vi "Telescope Read Current Status.vi"(8 "error in (no error)":errorcluster, 11 "PRIME Telescope in":refnum<class "PRIME Telescope.lvclass">) -> (0 "error out":errorcluster, 1 "Raw Response":string, 2 "Telescope Status":T1, 3 "PRIME Telescope out":refnum<class "PRIME Telescope.lvclass">, 4 "Cmd Sent":string="A 001 004 009 018 020 017\r")   [LabVIEW 2024, in "PRIME Telescope.lvclass"]
uses:
  PRIME Telescope.lvclass
  Telescope cluster Status.ctl
  typedefs/CC cluster RA and DEC.ctl
  Telescope enum Status.ctl
  PRIME Telescope.lvclass/PRIME Telescope.ctl
  Telescope.lvclass
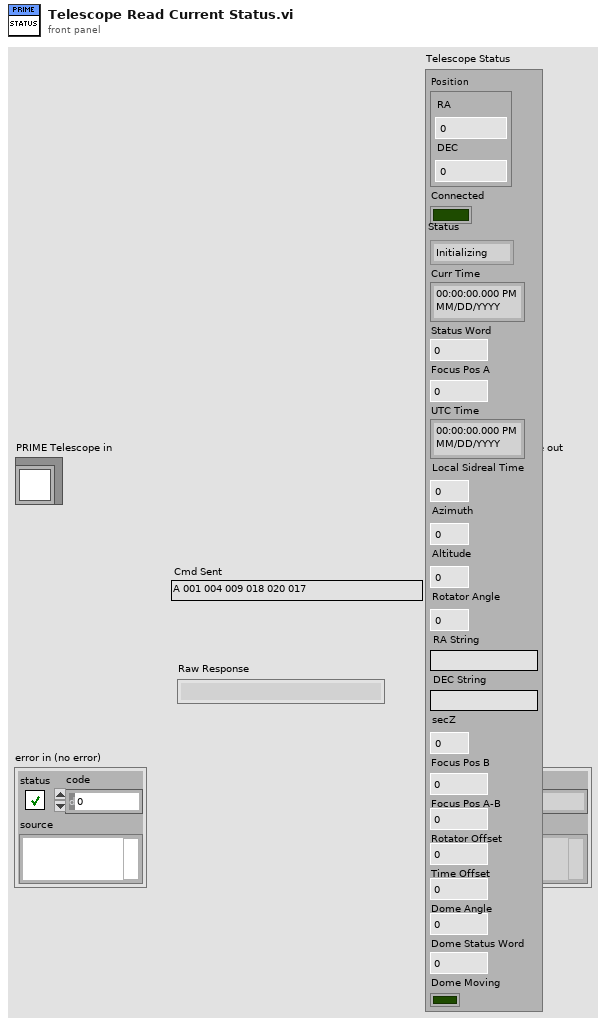
[diagram p1: front panel]
types:
  T1 = typedef "Telescope.lvclass/Telescope cluster Status.ctl" = cluster{"Position":T2, "Connected":bool, "Status":T3, "Curr Time":timestamp, "Status Word":u32, "Focus Pos A":dbl, "UTC Time":timestamp, "Local Sidreal Time":dbl, "Azimuth":dbl, "Altitude":dbl, "Rotator Angle":dbl, "RA String":string, "DEC String":string, "secZ":dbl, "Focus Pos B":dbl, "Focus Pos A-B":dbl, "Rotator Offset":dbl, "Time Offset":dbl, "Dome Angle":dbl, "Dome Status Word":u32, "Dome Moving":bool}
  T2 = typedef "CC cluster RA and DEC.ctl" = cluster{"RA":dbl, "DEC":dbl}
  T3 = typedef "Telescope.lvclass/Telescope enum Status.ctl" = enum16{"Initializing", "Ready", "Moving", "Focusing", "Error"}
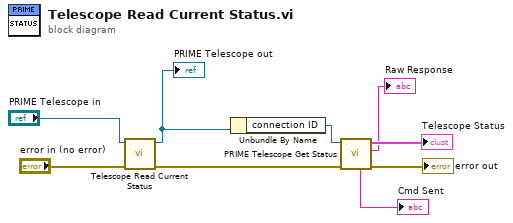
[diagram p0: block diagram]
diagram:
  n1 = call-parent "Telescope Read Current Status.vi"("error in (no error)"="error in (no error)", "Telescope in"="PRIME Telescope in") -> ("error out"=w5:errorcluster, "Telescope out"=w7:refnum<class "PRIME Telescope.lvclass">)  [unwired: 5 in, 3 out]
  "PRIME Telescope out" <- w7
  n2 = Unbundle By Name(w7) -> ("connection ID"=w6:refnum<k5>)
  n3 = call "PRIME Telescope Get Status.vi"("error in (no error)"=w5, "connection ID"=w6) -> ("error out"=→"error out":errorcluster, "Raw Response"=→"Raw Response":string, "Telescope Status"=→"Telescope Status":T1, "Cmd"=→"Cmd Sent":string)  [unwired: 5 in, 1 out]
